vi "packageTelemetrySnapshot.vi"(8 "Error In":errorcluster, 10 "All Data":T1 {"Power Readings"."Current" format="%#.3g A"; "Power Readings"."Power" format="%#.3g W"; "Power Readings"."Shunt Voltage" format=" %#.3g V"; "Power Readings"."Bus Voltage" format="%#.3g V"; "Power Readings"."Voltage (Total)" format="%#.3g V"; "ThermalReadings"."Ambient Temp (°F)" format="%.2f °F"; "ThermalReadings"."Ambient Temp (°C)" format="%.2f °C"; "ThermalReadings"."Object Temp (°F)" format="%.2f °F"; "ThermalReadings"."Object Temp (°C)" format="%.2f °C"; "CPU loads"."ISR (%)" format="%#.2f"; "CPU loads"."Idle (%)" format="%#.2f"; "CPU loads"."Background (%)" format="%#.2f"; "CPU loads"."Normal (%)" format="%#.2f"; "CPU loads"."Above Normal (%)" format="%#.2f"; "CPU loads"."High (%)" format="%#.2f"; "CPU loads"."Timed Structures (%)" format="%#.2f"; "CPU loads"."Time Critical (%)" format="%#.2f"; "CPU loads"."Total (%)" format="%#.2f"}, 11 "Send Non-Critical Data":bool) -> (0 "Error Out":errorcluster, 3 "Latest Critical Telemetry":T11)   [LabVIEW 2017]
uses:
  Type Defs/criticalTelemetry.ctl
  Type Defs/PodState.ctl
  Type Defs/allData.ctl
  Sensors/Power Sensor - Adafruit INA219/INA219 Measurements.ctl
  Type Defs/tempReadings.ctl
  Type Defs/AnalogPressureReading.ctl
  Type Defs/allLaserReadings.ctl
  Type Defs/laserReading.ctl
  Type Defs/tofReading.ctl
  <vilib>/Utility/RT CPU Load.ctl
  Type Defs/pressureReading.ctl
  <vilib>/NI_Real-Time Target Support.lvlib
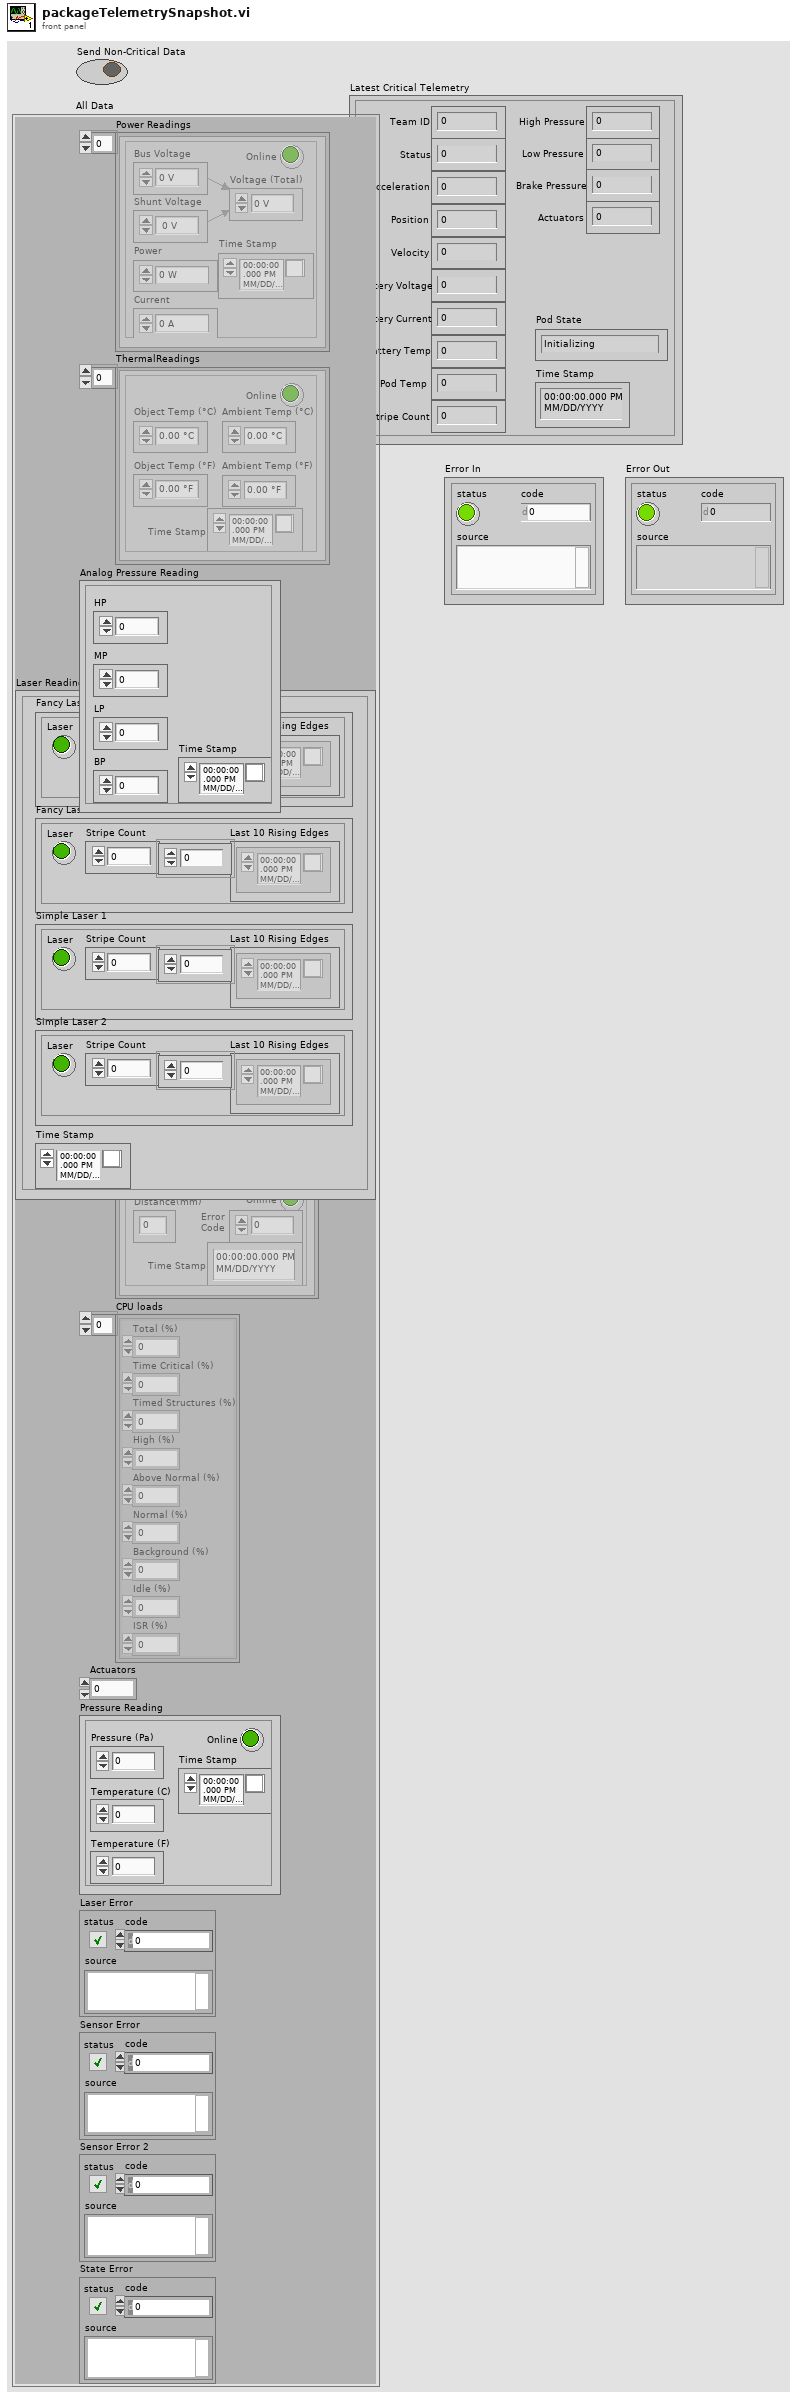
[diagram p1: front panel]
types:
  T1 = typedef "allData.ctl" = cluster{"Power Readings":T2[], "ThermalReadings":T3[], "Analog Pressure Reading":T4, "Laser Readings":T5, "Pod State":T7, "seconds since 1Jan1904":timestamp, "ToF Readings":T8[], "CPU loads":T9[], "Actuators":u32, "Pressure Reading":T10, "Laser Error":errorcluster, "Sensor Error":errorcluster, "Sensor Error 2":errorcluster, "State Error":errorcluster}
  T2 = typedef "INA219 Measurements.ctl" = cluster{"Voltage (Total)":dbl, "Bus Voltage":dbl, "Shunt Voltage":dbl, "Power":dbl, "Current":dbl, "Online":bool, "Time Stamp":timestamp}
  T3 = typedef "tempReadings.ctl" = cluster{"Object Temp (°C)":dbl, "Object Temp (°F)":dbl, "Ambient Temp (°C)":dbl, "Ambient Temp (°F)":dbl, "Online":bool, "Time Stamp":timestamp}
  T4 = typedef "AnalogPressureReading.ctl" = cluster{"HP":dbl, "MP":dbl, "LP":dbl, "BP":dbl, "Time Stamp":timestamp}
  T5 = typedef "allLaserReadings.ctl" = cluster{"Fancy Laser 1":T6, "Fancy Laser 2":T6, "Simple Laser 1":T6, "Simple Laser 2":T6, "Time Stamp":timestamp}
  T6 = typedef "laserReading.ctl" = cluster{"Laser":bool, "Stripe Count":u32, "Last 10 Rising Edges":timestamp[]}
  T7 = typedef "PodState.ctl" = enum16{"Initializing", "Pre-flight Testing", "Ready", "Pushing", "Coast", "Braking", "Post-flight", "Fault"}
  T8 = typedef "tofReading.ctl" = cluster{"Distance(mm)":u8, "Online":bool, "Error\nCode":u8, "Time Stamp":timestamp}
  T9 = typedef "NI_Real-Time Target Support.lvlib/RT CPU Load.ctl" = cluster{"Total (%)":dbl, "Time Critical (%)":dbl, "Timed Structures (%)":dbl, "High (%)":dbl, "Above Normal (%)":dbl, "Normal (%)":dbl, "Background (%)":dbl, "Idle (%)":dbl, "ISR (%)":dbl}
  T10 = typedef "pressureReading.ctl" = cluster{"Time Stamp":timestamp, "Online":bool, "Temperature (C)":dbl, "Pressure (Pa)":dbl, "Temperature (F)":dbl}
  T11 = typedef "criticalTelemetry.ctl" = cluster{"Team ID":u8, "Status":u8, "Acceleration":i32, "Position":i32, "Velocity":i32, "Battery Voltage":i32, "Battery Current":i32, "Battery Temp":i32, "Pod Temp":i32, "Stripe Count":u32, "High Pressure":dbl, "Low Pressure":dbl, "Brake Pressure":dbl, "Actuators":u32, "Pod State":T7, "Time Stamp":timestamp}
  T12 = typedef "positionData.ctl" = cluster{"Position (m)":dbl, "Velocity (m/s)":dbl, "Acceleration (m/s^2)":dbl}
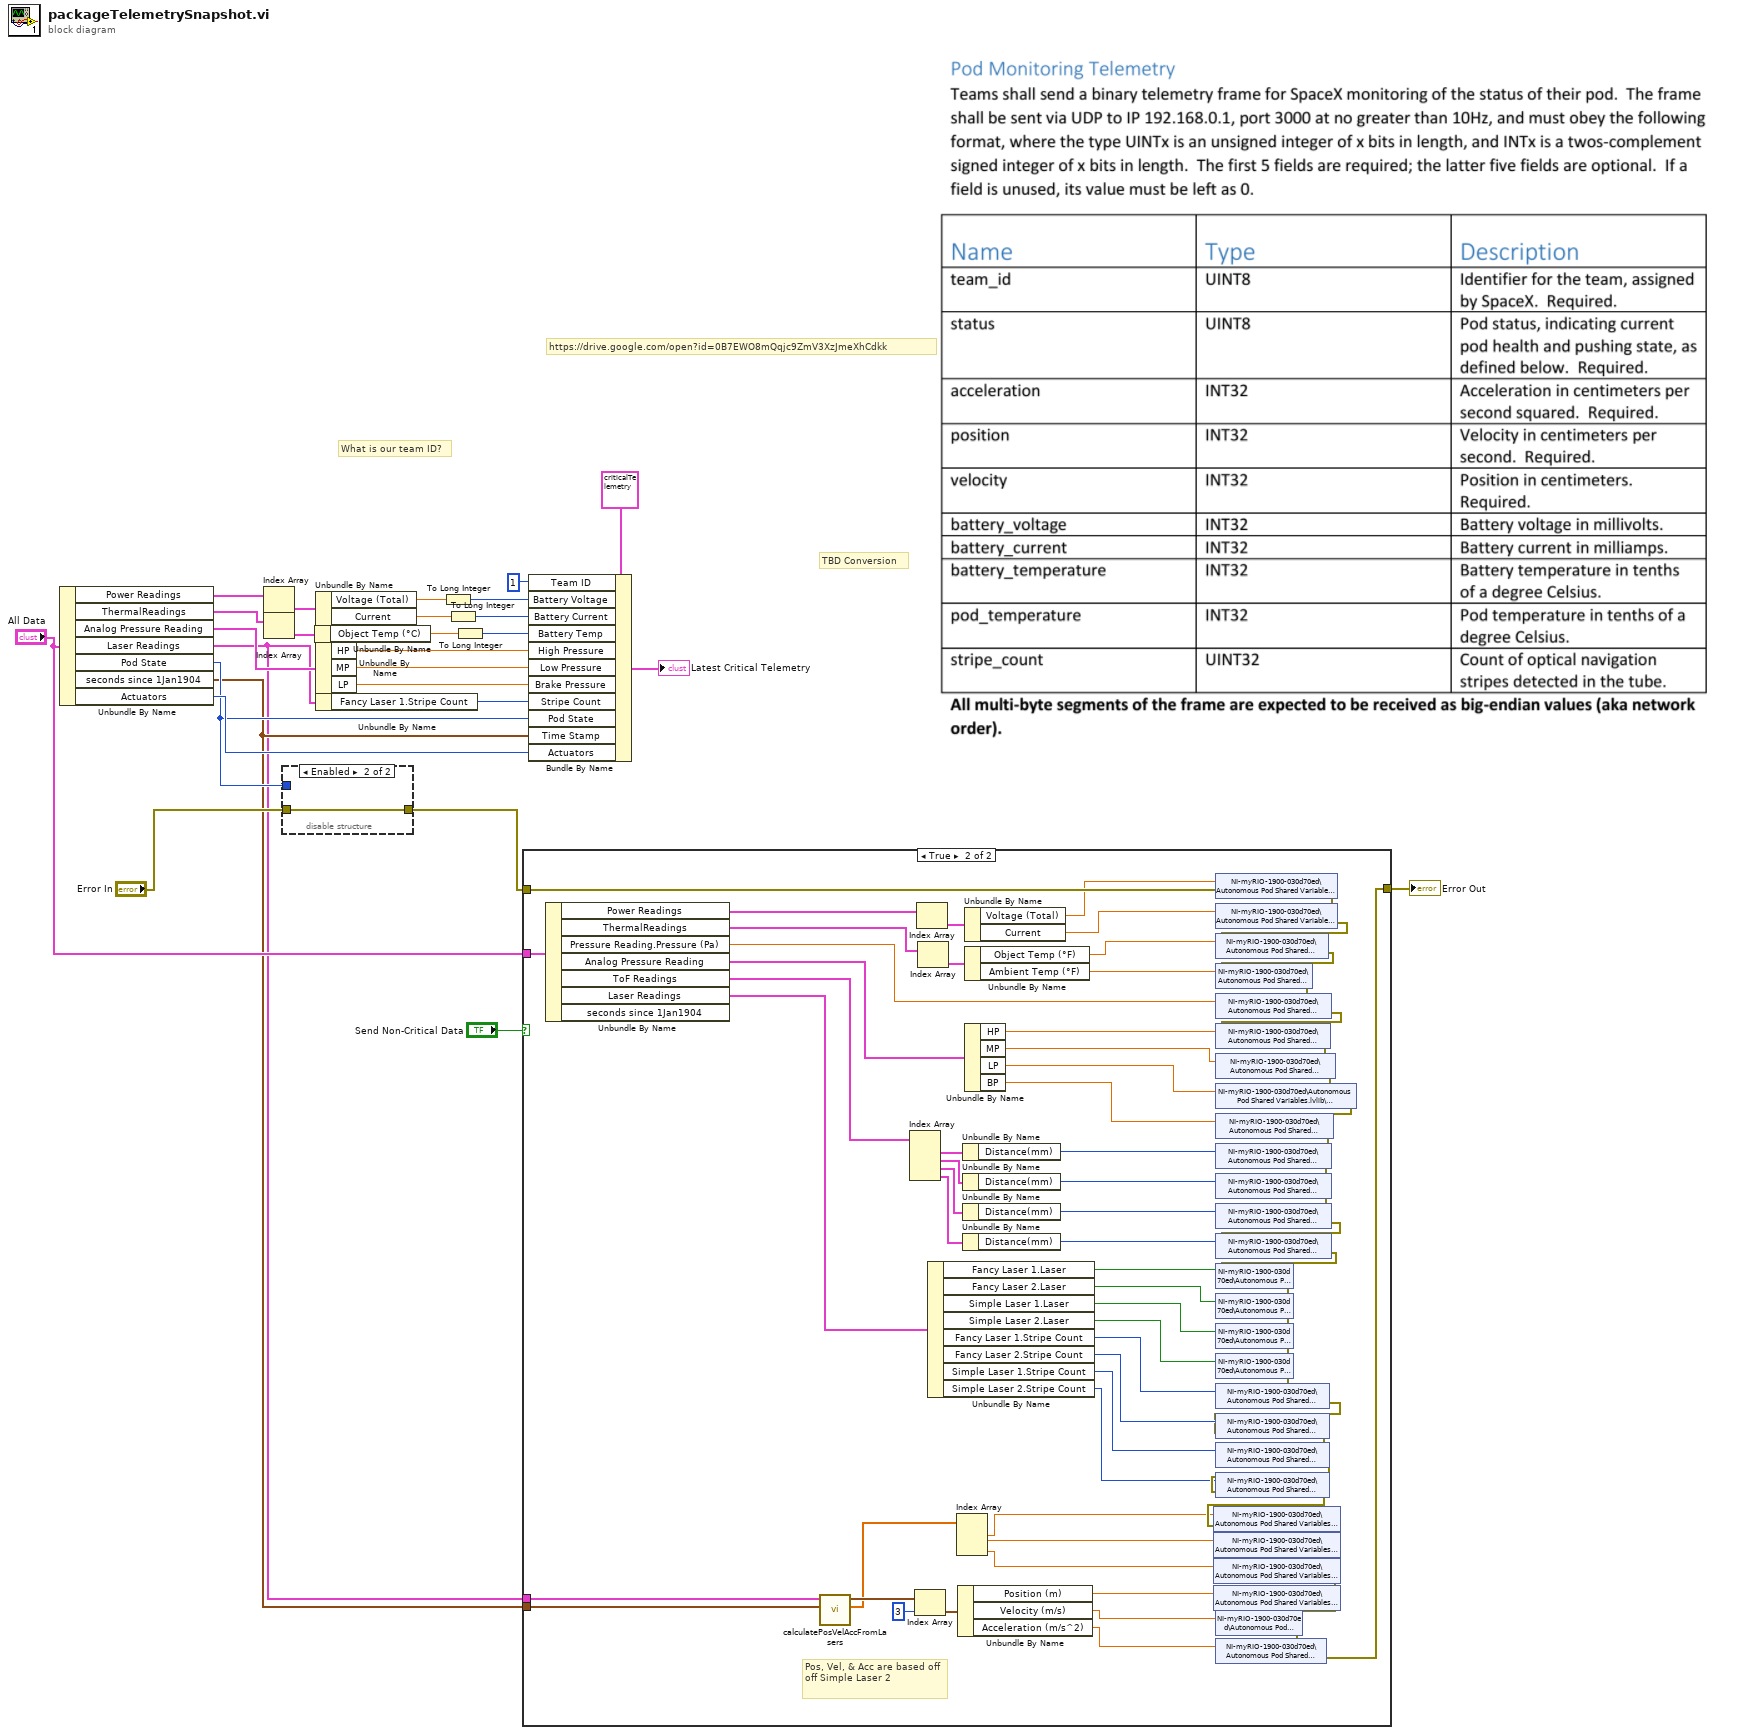
[diagram p0: block diagram]
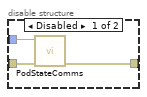
[diagram p2: hidden frame]
diagram:
  # "What is our team ID?"
  # "https://drive.google.com/open?id=0B7EWO8mQqjc9ZmV3XzJmeXhCdkk"
  # "TBD Conversion"
  n1 = Unbundle By Name("All Data") -> ("Power Readings"=w27:T2[], "ThermalReadings"=w22:T3[], "Analog Pressure Reading"=w19:T4, "Laser Readings"=w1:T5, "Pod State"=w5:T7, "seconds since 1Jan1904"=w2:timestamp, "Actuators"=w6:u32)
  n2 = Index Array(array=w27) -> (element=w25:T2)  [unwired: 1 in]
  n3 = Index Array(array=w22) -> (element=w21:T3)  [unwired: 1 in]
  n4 = disable-structure shown="Enabled" {
    disable-tunnel: w5 -> [w30 _]
    disable-tunnel: "Error In" -> [w29 w31]
    disable-tunnel: [w28 w31] -> w3
    frame Disabled {
      n5 = call "PodStateComms.vi"("error in"=w29, "Pod State"=w30) -> ("error out"=w28:errorcluster)  [unwired: 9 in]
    }
    frame Enabled {
    }
  }
  n6 = Unbundle By Name(w21) -> ("Object Temp (°C)"=w20:dbl)
  n7 = Unbundle By Name(w25) -> ("Voltage (Total)"=w24:dbl, "Current"=w23:dbl)
  n8 = Unbundle By Name(w19) -> ("HP"=w18:dbl, "MP"=w17:dbl, "LP"=w16:dbl)
  n9 = Unbundle By Name(w1) -> ("Fancy Laser 1.Stripe Count"=w13:u32)
  n10 = To Long Integer(number=w24) -> (32bit integer=w12:i32)
  n11 = To Long Integer(number=w23) -> (32bit integer=w11:i32)
  n12 = To Long Integer(number=w20) -> (32bit integer=w10:i32)
  n13 = case shown="True" "Send Non-Critical Data" {
    tunnel: "All Data" -> [_ w100]
    tunnel: w3 -> [w32 w99]
    tunnel: [w32 w41] -> w7
    tunnel: w2 -> [_ w49]
    tunnel: w1 -> [_ w48]
    frame False {
    }
    frame True {
      # "Pos, Vel, & Acc are based off off Simple Laser 2"
      n14 = Unbundle By Name(w100) -> ("Power Readings"=w101:T2[], "ThermalReadings"=w103:T3[], "Pressure Reading.Pressure (Pa)"=w94:dbl, "Analog Pressure Reading"=w105:T4, "ToF Readings"=w89:T8[], "Laser Readings"=w80:T5)  [unwired: 1 out]
      n15 = call "calculatePosVelAccFromLasers.vi"("Right Now"=w49, "Laser Readings"=w48) -> ("Positions"=w36:dbl[], "Position Calculations"=w47:T12[])  [unwired: 8 in]
      n16 = Index Array(array=w89) -> (element #1=w88:T8, element #2=w81:T8, element #3=w82:T8, element #4=w83:T8)  [unwired: 4 in]
      n17 = Index Array(array=w47, index=3) -> (element=w45:T12)
      n18 = Index Array(array=w101) -> (element=w102:T2)  [unwired: 1 in]
      n19 = Index Array(array=w103) -> (element=w104:T3)  [unwired: 1 in]
      n20 = Unbundle By Name(w80) -> ("Fancy Laser 1.Laser"=w79:bool, "Fancy Laser 2.Laser"=w78:bool, "Simple Laser 1.Laser"=w77:bool, "Simple Laser 2.Laser"=w76:bool, "Fancy Laser 1.Stripe Count"=w75:u32, "Fancy Laser 2.Stripe Count"=w74:u32, "Simple Laser 1.Stripe Count"=w53:u32, "Simple Laser 2.Stripe Count"=w52:u32)
      n21 = Index Array(array=w36) -> (element #1=w35:dbl, element #2=w34:dbl, element #3=w33:dbl)  [unwired: 3 in]
      n22 = Unbundle By Name(w45) -> ("Position (m)"=w44:dbl, "Velocity (m/s)"=w43:dbl, "Acceleration (m/s^2)"=w42:dbl)
      n23 = Unbundle By Name(w88) -> ("Distance(mm)"=w87:u8)
      n24 = Unbundle By Name(w81) -> ("Distance(mm)"=w84:u8)
      n25 = Unbundle By Name(w82) -> ("Distance(mm)"=w85:u8)
      n26 = Unbundle By Name(w83) -> ("Distance(mm)"=w86:u8)
      n27 = Unbundle By Name(w102) -> ("Voltage (Total)"=w98:dbl, "Current"=w97:dbl)
      n28 = Unbundle By Name(w104) -> ("Object Temp (°F)"=w96:dbl, "Ambient Temp (°F)"=w95:dbl)
      n29 = Unbundle By Name(w105) -> ("HP"=w93:dbl, "MP"=w92:dbl, "LP"=w91:dbl, "BP"=w90:dbl)
      n30 = shared-variable "NI-myRIO-1900-030d70ed\\Autonomous Pod Shared Variables.lvlib\\BatteryVoltage"(w98, error in=w99) -> (error out=w73:errorcluster)
      n31 = shared-variable "NI-myRIO-1900-030d70ed\\Autonomous Pod Shared Variables.lvlib\\BatteryCurrent"(w97, error in=w73) -> (error out=w72:errorcluster)
      n32 = shared-variable "NI-myRIO-1900-030d70ed\\Autonomous Pod Shared Variables.lvlib\\BatteryTemp"(w96, error in=w72) -> (error out=w71:errorcluster)
      n33 = shared-variable "NI-myRIO-1900-030d70ed\\Autonomous Pod Shared Variables.lvlib\\PodTemp"(w95, error in=w71) -> (error out=w70:errorcluster)
      n34 = shared-variable "NI-myRIO-1900-030d70ed\\Autonomous Pod Shared Variables.lvlib\\TubePressure"(w94, error in=w70) -> (error out=w69:errorcluster)
      n35 = shared-variable "NI-myRIO-1900-030d70ed\\Autonomous Pod Shared Variables.lvlib\\HighPressure"(w93, error in=w69) -> (error out=w68:errorcluster)
      n36 = shared-variable "NI-myRIO-1900-030d70ed\\Autonomous Pod Shared Variables.lvlib\\UtilityPressure"(w92, error in=w68) -> (error out=w67:errorcluster)
      n37 = shared-variable "NI-myRIO-1900-030d70ed\\Autonomous Pod Shared Variables.lvlib\\LevitationPressure"(w91, error in=w67) -> (error out=w66:errorcluster)
      n38 = shared-variable "NI-myRIO-1900-030d70ed\\Autonomous Pod Shared Variables.lvlib\\BrakePressure"(w90, error in=w66) -> (error out=w65:errorcluster)
      n39 = shared-variable "NI-myRIO-1900-030d70ed\\Autonomous Pod Shared Variables.lvlib\\ToF1Distance"(w87, error in=w65) -> (error out=w64:errorcluster)
      n40 = shared-variable "NI-myRIO-1900-030d70ed\\Autonomous Pod Shared Variables.lvlib\\ToF2Distance"(w84, error in=w64) -> (error out=w63:errorcluster)
      n41 = shared-variable "NI-myRIO-1900-030d70ed\\Autonomous Pod Shared Variables.lvlib\\ToF3Distance"(w85, error in=w63) -> (error out=w62:errorcluster)
      n42 = shared-variable "NI-myRIO-1900-030d70ed\\Autonomous Pod Shared Variables.lvlib\\ToF4Distance"(w86, error in=w62) -> (error out=w61:errorcluster)
      n43 = shared-variable "NI-myRIO-1900-030d70ed\\Autonomous Pod Shared Variables.lvlib\\Laser1"(w79, error in=w61) -> (error out=w60:errorcluster)
      n44 = shared-variable "NI-myRIO-1900-030d70ed\\Autonomous Pod Shared Variables.lvlib\\Laser2"(w78, error in=w60) -> (error out=w59:errorcluster)
      n45 = shared-variable "NI-myRIO-1900-030d70ed\\Autonomous Pod Shared Variables.lvlib\\Laser3"(w77, error in=w59) -> (error out=w58:errorcluster)
      n46 = shared-variable "NI-myRIO-1900-030d70ed\\Autonomous Pod Shared Variables.lvlib\\Laser4"(w76, error in=w58) -> (error out=w57:errorcluster)
      n47 = shared-variable "NI-myRIO-1900-030d70ed\\Autonomous Pod Shared Variables.lvlib\\StripeCount1"(w75, error in=w57) -> (error out=w56:errorcluster)
      n48 = shared-variable "NI-myRIO-1900-030d70ed\\Autonomous Pod Shared Variables.lvlib\\StripeCount2"(w74, error in=w56) -> (error out=w55:errorcluster)
      n49 = shared-variable "NI-myRIO-1900-030d70ed\\Autonomous Pod Shared Variables.lvlib\\StripeCount3"(w53, error in=w55) -> (error out=w54:errorcluster)
      n50 = shared-variable "NI-myRIO-1900-030d70ed\\Autonomous Pod Shared Variables.lvlib\\StripeCount4"(w52, error in=w54) -> (error out=w40:errorcluster)
      n51 = shared-variable "NI-myRIO-1900-030d70ed\\Autonomous Pod Shared Variables.lvlib\\PositionFLaser1"(w35, error in=w40) -> (error out=w39:errorcluster)
      n52 = shared-variable "NI-myRIO-1900-030d70ed\\Autonomous Pod Shared Variables.lvlib\\PositionFLaser2"(w34, error in=w39) -> (error out=w38:errorcluster)
      n53 = shared-variable "NI-myRIO-1900-030d70ed\\Autonomous Pod Shared Variables.lvlib\\PositionSLaser1"(w33, error in=w38) -> (error out=w37:errorcluster)
      n54 = shared-variable "NI-myRIO-1900-030d70ed\\Autonomous Pod Shared Variables.lvlib\\PositionSLaser2"(w44, error in=w37) -> (error out=w51:errorcluster)
      n55 = shared-variable "NI-myRIO-1900-030d70ed\\Autonomous Pod Shared Variables.lvlib\\Velocity"(w43, error in=w51) -> (error out=w50:errorcluster)
      n56 = shared-variable "NI-myRIO-1900-030d70ed\\Autonomous Pod Shared Variables.lvlib\\Acceleration"(w42, error in=w50) -> (error out=w41:errorcluster)
    }
  }
  "Error Out" <- w7
  n57 = Bundle By Name(cluster=T11 {"Team ID"=0, "Status"=0, "Acceleration"=0, "Position"=0, "Velocity"=0, "Battery Voltage"=0, "Battery Current"=0, "Battery Temp"=0, "Pod Temp"=0, "Stripe Count"=0, "High Pressure"=0.0, "Low Pressure"=0.0, "Brake Pressure"=0.0, "Actuators"=0, "Pod State"=enum."Initializing", "Time Stamp"=timestamp(0 s since 1904-01-01)} ("Latest Critical Telemetry"), "Team ID"=u8 1, "Battery Voltage"=w12, "Battery Current"=w11, "Battery Temp"=w10, "High Pressure"=w18, "Low Pressure"=w17, "Brake Pressure"=w16, "Stripe Count"=w13, "Pod State"=w5, "Time Stamp"=w2, "Actuators"=w6) -> (→"Latest Critical Telemetry":T11)
